vi "Write Numeric Text.vi"(5 "NumericText":refnum<class "NumericText.lvclass">, 9 "Digital in":refnum<class "Digital.lvclass">) -> (3 "Digital out":refnum<class "Digital.lvclass">)   [LabVIEW 2014, in "Digital.lvclass"]
uses:
  Digital.lvclass
  NumericText/NumericText.lvclass
  Digital.lvclass/Digital.ctl
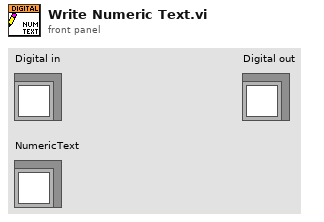
[diagram p1: front panel]
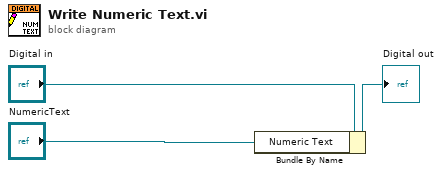
[diagram p0: block diagram]
diagram:
  n1 = Bundle By Name(cluster="Digital in", "Numeric Text"="NumericText") -> (→"Digital out":refnum<class "Digital.lvclass">)
